vi "Add SR Popup.vi"(8 "error in":errorcluster, 11 "SR number array in":i32[](array[numeric])) -> (0 "error out":errorcluster, 3 "SR number array out":i32[](array[numeric]))   [LabVIEW 2018]
uses:
  <vilib>/Utility/miscctls.llb/LVPointTypeDef.ctl
panel:
  in  "Close":bool
  in  "Add SR":bool
  in  "SR to Add":i32
  # "Enter SR number and press\n\"Add SR\" to add it to the list"
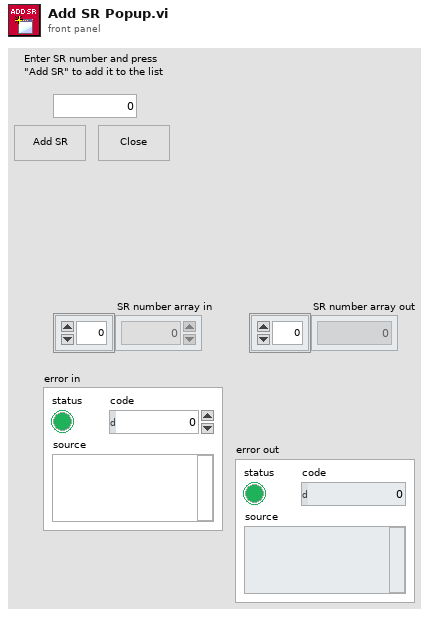
[diagram p1: front panel]
types:
  T1 = typedef "LVPointTypeDef.ctl" = cluster{"Horizontal":i16, "Vertical":i16}
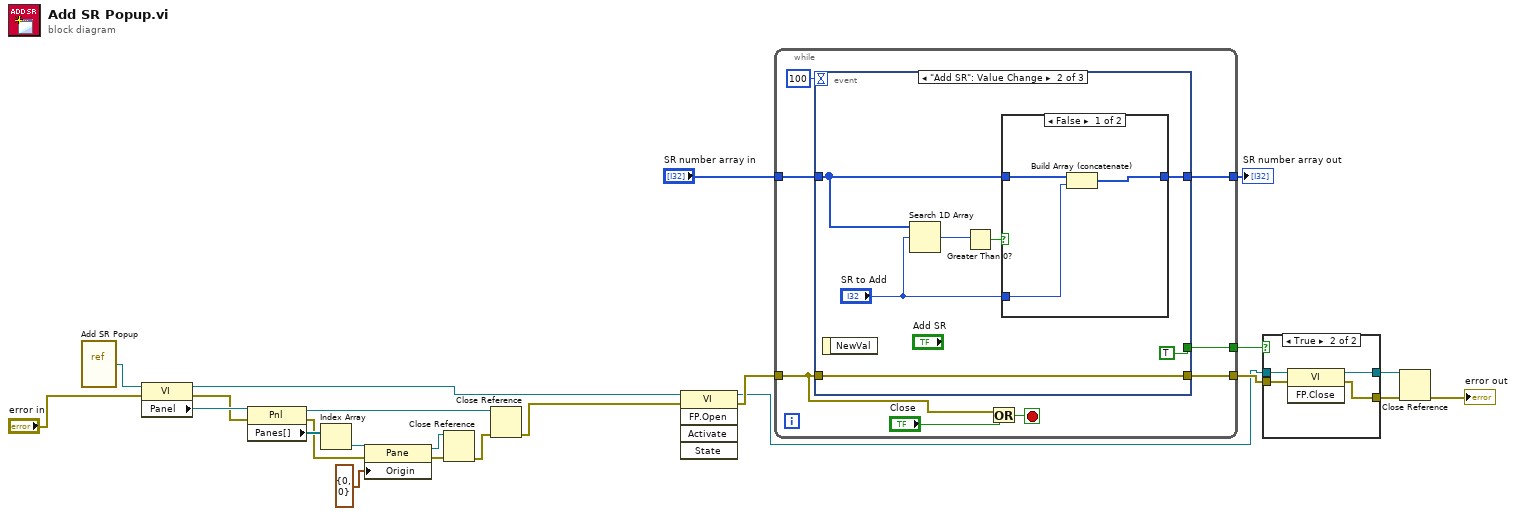
[diagram p0: block diagram]
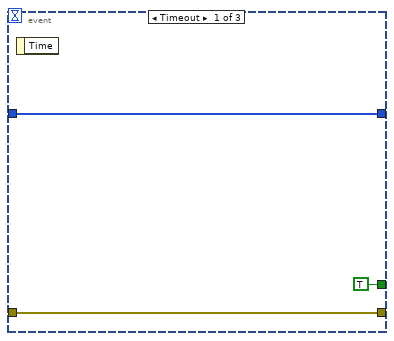
[diagram p3: hidden frame]
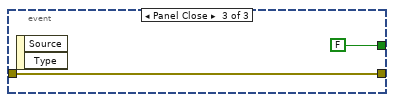
[diagram p5: hidden frame]
diagram:
  n1 = vi-ref "Add SR Popup.vi"() -> (w21:refnum<vi>)
  n2 = property class="VI"(reference=w21, error in="error in") -> (reference out=w3:refnum<vi>, error out=w11:errorcluster, "Panel"=w12:refnum<vi>)
  n3 = property class="Pnl"(reference=w12, error in=w11) -> (reference out=w13:refnum<vi>, error out=w18:errorcluster, "Panes[]"=w20:refnum<vi>[])
  n4 = Index Array(array=w20) -> (element=w19:refnum<vi>)  [unwired: 1 in]
  n5 = property class="Pane"(reference=w19, error in=w18, "Origin"=T1 {"Horizontal"=0, "Vertical"=0}) -> (reference out=w16:refnum<vi>, error out=w15:errorcluster)
  n6 = Close Reference(reference=w16, error in (no error)=w15) -> (error out=w14:errorcluster)
  n7 = Close Reference(reference=w13, error in (no error)=w14) -> (error out=w2:errorcluster)
  n8 = invoke class="VI" method="FP.Open"(reference=w3, error in=w2) -> (reference out=w4:refnum<vi>, error out=w10:errorcluster)  [unwired: 3 in, 3 out]
  n9 = while {
    tunnel: "SR number array in" -> [w31]
    tunnel: [w30] -> w22
    tunnel: w10 -> [w24]
    tunnel: [w28] -> w9
    tunnel: [w27] -> w8
    stop <- w26 stop-if-true
    n10 = event shown="[1] \"Add SR\": Value Change" {
      selector: _ -> [_ _ _]
      dyn-events: _ -> [_ _ _]
      timeout: 100 -> [_ _ _]
      tunnel: w31 -> [w34 w40 _]
      tunnel: [w34 w38 _] -> w30
      tunnel: w24 -> [w32 w36 w46]
      tunnel: [w32 w36 w46] -> w28
      tunnel: [TRUE TRUE FALSE] -> w27
      event Timeout {
        n11 = event-data() -> ()  [unwired: 1 in, 1 out]
      }
      event "Add SR": Value Change {
        n12 = event-data() -> ()  [unwired: 1 in, 1 out]
        n13 = Search 1D Array(1D array=w40, element="SR to Add") -> (index of element=w39:i32)  [unwired: 1 in]
        n14 = Greater Than 0?(x=w39) -> (x > 0?=w41:bool)
        n15 = case shown="False" w41 {
          tunnel: w40 -> [w44 w45]
          tunnel: [w43 w45] -> w38
          tunnel: "SR to Add" -> [w42 _]
          frame False {
            n16 = Build Array (concatenate)(w44, w42) -> (w43:i32[])
          }
          frame True {
          }
        }
      }
      event Panel Close {
        n17 = event-data() -> ()  [unwired: 1 in, 2 out]
      }
    }
    n18 = Or(x=w24, y="Close") -> (x .or. y?=w26:bool)
  }
  "SR number array out" <- w22
  n19 = case shown="True" w8 {
    tunnel: w4 -> [w49 w53]
    tunnel: w9 -> [w48 w52]
    tunnel: [w49 w51] -> w7
    tunnel: [w48 w50] -> w6
    frame False {
    }
    frame True {
      n20 = invoke class="VI" method="FP.Close"(reference=w53, error in=w52) -> (reference out=w51:refnum<vi>, error out=w50:errorcluster)  [unwired: 1 in, 1 out]
    }
  }
  n21 = Close Reference(reference=w7, error in (no error)=w6) -> (error out=→"error out":errorcluster)
